vi "create.OrderExecuted.vi"(8 "error in":errorcluster, 10 "OrderExecuted.Parameters":T1, 11 "OrderExecuted in":refnum<class "OrderExecuted.lvclass">) -> (0 "error out":errorcluster, 3 "OrderExecuted out":refnum<class "OrderExecuted.lvclass">)   [LabVIEW 2020, in "OrderExecuted.lvclass"]
uses:
  OrderExecuted.lvclass
  OrderExecuted.Parameters.ctl
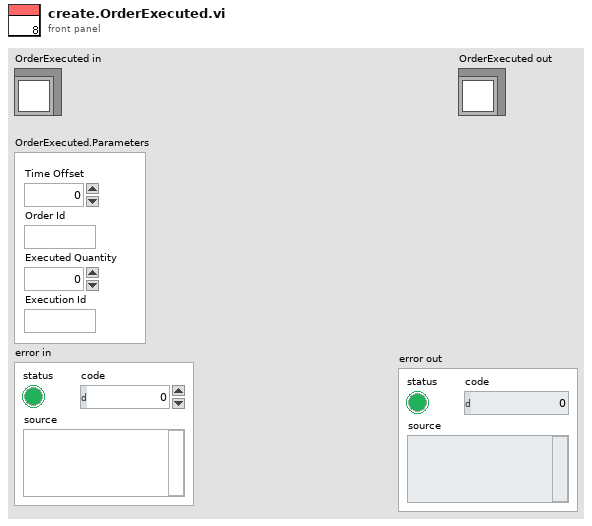
[diagram p1: front panel]
types:
  T1 = typedef "OrderExecuted.lvclass/OrderExecuted.Parameters.ctl" = cluster{"Time Offset":u32, "Order Id":string, "Executed Quantity":u32, "Execution Id":string}
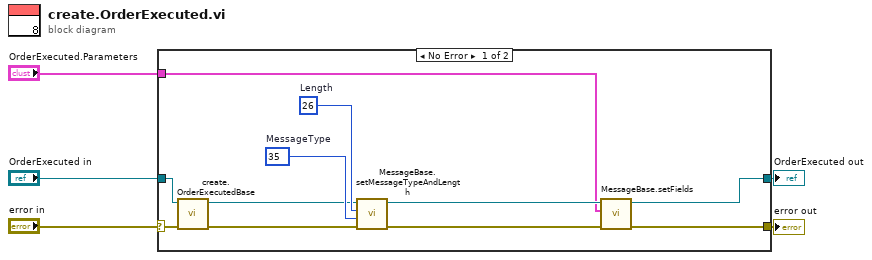
[diagram p0: block diagram]
diagram:
  n1 = case shown="No Error" "error in" {
    selector: "error in" -> [w9 w18]
    tunnel: [w7 w18] -> w2
    tunnel: [w6 w17] -> w4
    tunnel: "OrderExecuted in" -> [w10 w17]
    tunnel: "OrderExecuted.Parameters" -> [w8 _]
    frame No Error {
      w15 = u8 35  # MessageType
      w16 = u8 26  # Length
      n2 = call-dynamic "create.OrderExecutedBase.vi"("error in (no error)"=w9, "OrderExecutedBase in"=w10) -> ("error out"=w14:errorcluster, "OrderExecutedBase out"=w13:refnum<class "OrderExecuted.lvclass">)  [unwired: 8 in]
      n3 = call-dynamic "MessageBase.setMessageTypeAndLength.vi"("error in (no error)"=w14, "MessageType"=w15, "Length"=w16, "MessageBase in"=w13) -> ("error out"=w11:errorcluster, "MessageBase out"=w12:refnum<class "OrderExecuted.lvclass">)  [unwired: 6 in]
      n4 = call-dynamic "MessageBase.setFields.vi"("error in (no error)"=w11, "Cluster (dup)"=w8, "MessageBase in"=w12) -> ("error out"=w7:errorcluster, "MessageBase out"=w6:refnum<class "OrderExecuted.lvclass">)  [unwired: 7 in]
    }
    frame Error {
    }
  }
  "OrderExecuted out" <- w4
  "error out" <- w2
